vi "VIS-IR_INIT-drv.vi"(8 "error in (no error)":errorcluster, 11 "VIS-IR in":refnum<class "VIS-NIR.lvclass">) -> (0 "error out":errorcluster, 3 "VIS-IR out":refnum<class "VIS-NIR.lvclass">)   [LabVIEW 2015, in "VIS-NIR.lvclass"]
uses:
  VIS-NIR.lvclass
  dependecies/ControlsVIs/Clusters-def/list-of-DAQmx-tasks.ctl
  dependecies/ControlsVIs/Clusters-def/list-of-keys-DAQmx-tasks.ctl
  GeneralFunctionality/GeneralFunctionality.lvclass/GeneralFunctionality.ctl
  Detector.lvclass/Detector.ctl
  dependecies/globalVarII.vi
  Config/Config.lvclass
  Detector.lvclass
  DAQmxTasks/DAQmxTaskContainer_General/DAQmxTaksContainer_General.lvclass
  GeneralFunctionality/GeneralFunctionality.lvclass
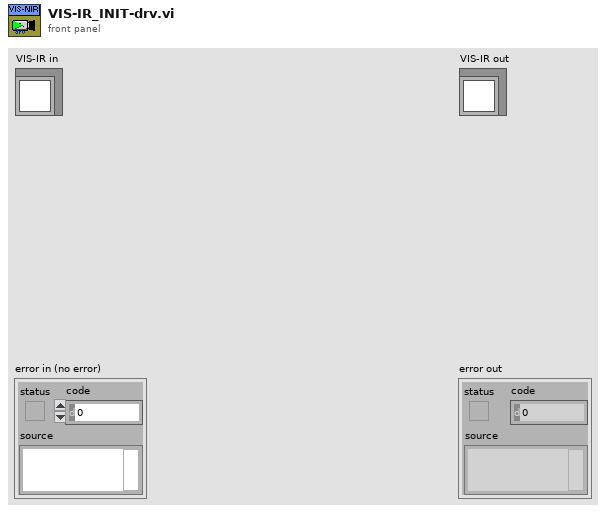
[diagram p1: front panel]
types:
  T1 = typedef "DAQmxTaksContainer_General.lvclass/list-of-keys-DAQmx-tasks.ctl" = string
  T2 = typedef "DAQmxTaksContainer_General.lvclass/list-of-DAQmx-tasks.ctl" = string
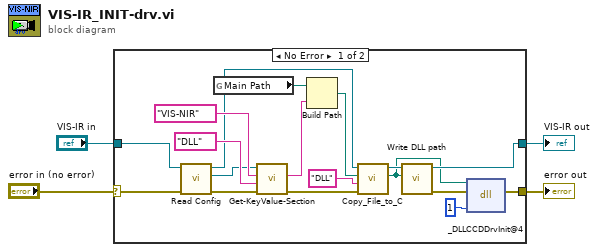
[diagram p0: block diagram]
diagram:
  n1 = case shown="No Error" "error in (no error)" {
    selector: "error in (no error)" -> [w13 w24]
    tunnel: [w12 w24] -> w3
    tunnel: [w11 w23] -> w1
    tunnel: "VIS-IR in" -> [w14 w23]
    frame No Error {
      n2 = call "Read Config.vi"("error in (no error)"=w13, "GeneralFunctionality en entrée"=w14) -> ("error out"=w16:errorcluster, "Config.lvclass"=w17:refnum<class "Config.lvclass">, "GeneralFunctionality en sortie"=w10:refnum<class "VIS-NIR.lvclass">)  [unwired: 7 in]
      n3 = global read "globalVarII.vi" "Main Path"() -> (w18:path)
      n4 = call-dynamic "Get-KeyValue-Section.vi"("error in (no error)"=w16, "Key"=T1 "DLL", "Section"=T2 "VIS-NIR", "Config in"=w17) -> ("error out"=w8:errorcluster, "Value"=w19:string)  [unwired: 5 in, 1 out]
      n5 = Build Path(base path=w18, name or relative path=w19) -> (appended path=w7:path)
      n6 = call "Copy_File_to_C.vi"("error in (no error)"=w8, "Folder"="DLL", "path from"=w7, "GeneralFunctionality in"=w10) -> ("appended path out"=w5:path, "GeneralFunctionality out"=w9:refnum<class "VIS-NIR.lvclass">)  [unwired: 5 in, 1 out]
      n7 = call "Write DLL path.vi"("DLL path"=w5, "Detector in"=w9) -> ("error out"=w22:errorcluster, "Detector out"=w11:refnum<class "VIS-NIR.lvclass">)  [unwired: 8 in]
      n8 = dll-call lib="G:/SD/TRANCON/DLL/ESLSCDLL.dll" fn="_DLLCCDDrvInit@4" ("lwlscdll.dll:DLLCCDDrvInit")(path in=w5, error in=w22, "drv"=u32 1) -> (error out=w12:errorcluster)  [unwired: 3 in, 1 out]
    }
    frame Error {
    }
  }
  "error out" <- w3
  "VIS-IR out" <- w1
